vi "Pass Fail Dialog.vi"(8 "error in (no error)":errorcluster, 11 "Pass/Fail":bool) -> (0 "error out":errorcluster)   [LabVIEW 2020]
doc: "Selection is true if Yes was pressed or on timeout. Selection is false only if No was pressed before timeout."
panel:
  in  "ok":bool
  out "Message":string
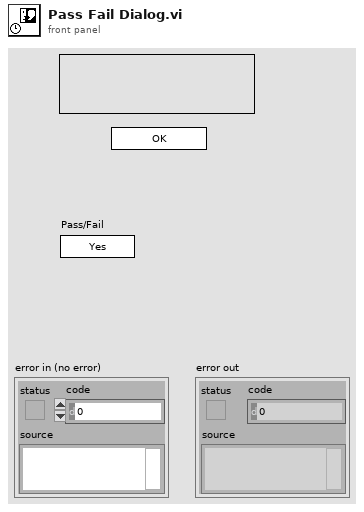
[diagram p1: front panel]
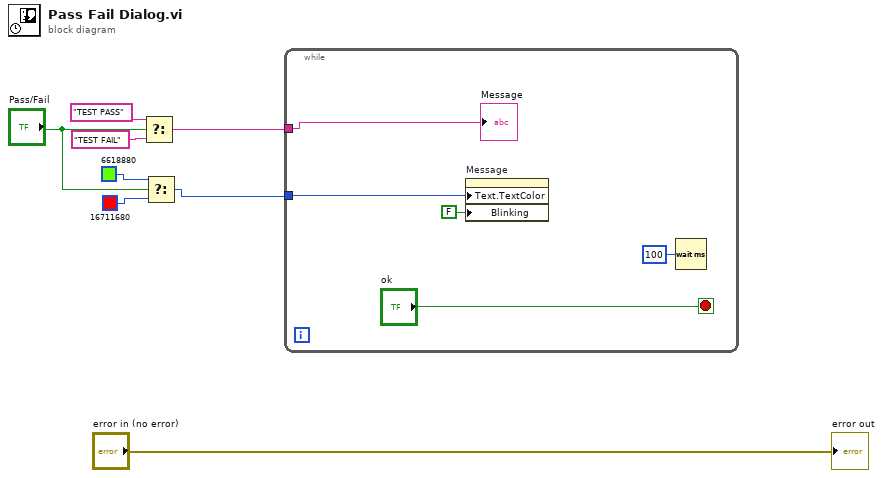
[diagram p0: block diagram]
diagram:
  n1 = Select(t="TEST PASS", s="Pass/Fail", f="TEST FAIL") -> (s? t:f=w5:string)
  n2 = Select(t=u32 6618880 ("Text.Text Colors:BG Color"), s="Pass/Fail", f=u32 16711680 ("Text.Text Colors:BG Color")) -> (s? t:f=w3:u32)
  n3 = while {
    tunnel: w5 -> [w13]
    tunnel: w3 -> [w10]
    stop <- "ok" stop-if-true
    n4 = property on="Message" class="Str"("Text.TextColor"=w10, "Blinking"=FALSE) -> ()  [unwired: 2 in, 2 out]
    n5 = Wait (ms)(milliseconds to wait=u32 100) -> ()  [unwired: 1 out]
    "Message" <- w13
  }
  "error out" <- "error in (no error)"
